vi "Go Back.vi"(0 "Display State In":T1={"WebView2 Ref"=refnum, "event callback refnum"=refnum, "Events"={"Navigation Complete Event"=refnum, "Source Changed Event"=refnum, "Document Title Changed Event"=refnum, "Status Bar Text Changed"=refnum, "Web Message Received"=refnum, "Window Close Requested"=refnum}, "Paths"={"Webview2 Native"=path "C:/Users/kleins/Desktop/webview2/microsoft.web.webview2.1.0.1370.28/build/native", "Edge Application"=path "", "User Data"=path ""}}, 9 "Container State":T3, 11 "error in (no error)":errorcluster) -> (4 "Display State Out":T1={"WebView2 Ref"=refnum, "event callback refnum"=refnum, "Events"={"Navigation Complete Event"=refnum, "Source Changed Event"=refnum, "Document Title Changed Event"=refnum, "Status Bar Text Changed"=refnum, "Web Message Received"=refnum, "Window Close Requested"=refnum}, "Paths"={"Webview2 Native"=path "C:/Users/kleins/Desktop/webview2/microsoft.web.webview2.1.0.1370.28/build/native", "Edge Application"=path "", "User Data"=path ""}}, 15 "error out":errorcluster)   [LabVIEW 2020, in "WebView2 Control.xctl"]
uses:
  WebView2 Control.xctl
  <vilib>/_xctls/Container State.ctl
  State.ctl
  C:/Users/kleins/Desktop/webview2/microsoft.web.webview2.1.0.1370.28/lib/net45/Microsoft.Web.WebView2.WinForms.dll
  microsoft.web.webview2.1.0.1370.28/lib/net45/Microsoft.Web.WebView2.WinForms.dll
  Paths.ctl
  <vilib>/_xctls/XControlSupport.lvlib
panel:
  # "Add Controls & Indicators that form the parameters of the method here. Hook them to the connector pane. Do not delete the controls & indicators that are already hooked to the connector pane.\n \nTo setup the parameters  for this method, right click on this item in the Project Tree & select \"Configure Method...\"."
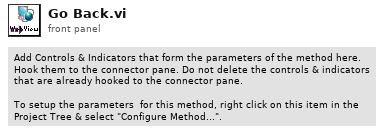
[diagram p1: front panel]
types:
  T1 = typedef "WebView2 Control.xctl/State.ctl" = cluster{"WebView2 Ref":refnum<data-value>, "event callback refnum":refnum<k27>, "Events":cluster{"Navigation Complete Event":refnum<user-event>, "Source Changed Event":refnum<user-event>, "Document Title Changed Event":refnum<user-event>, "Status Bar Text Changed":refnum<user-event>, "Web Message Received":refnum<user-event>, "Window Close Requested":refnum<user-event>}, "Paths":T2}
  T2 = typedef "WebView2 Control.xctl/Paths.ctl" = cluster{"Webview2 Native":path, "Edge Application":path, "User Data":path}
  T3 = typedef "XControlSupport.lvlib/Container State.ctl" = cluster{"Indicator?":bool, "Run Mode?":bool, " Refnum":refnum<vi>}
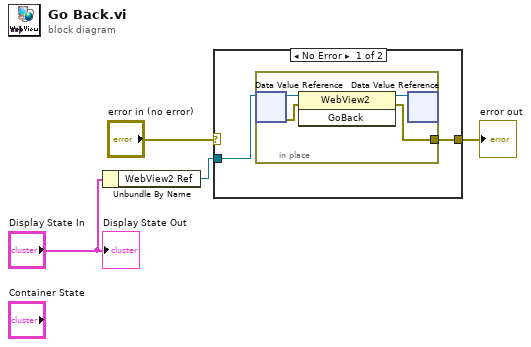
[diagram p0: block diagram]
diagram:
  n1 = Unbundle By Name("Display State In") -> ("WebView2 Ref"=w3:refnum<data-value>)
  n2 = case shown="No Error" "error in (no error)" {
    selector: "error in (no error)" -> [_ w11]
    tunnel: [w6 w11] -> w1
    tunnel: w3 -> [w5 _]
    frame No Error {
      n3 = in-place {
        in-place-border: [w10] -> w6
        n4 = in-place-dvr #1(w5) -> (w9:refnum<k24>, w8:errorcluster)
        n5 = invoke class="WebView2" method="GoBack"(reference=w9, error in=w8) -> (reference out=w7:refnum<k24>, error out=w10:errorcluster)  [unwired: 1 in, 1 out]
        n6 = in-place-dvr #1(w7) -> ()  [unwired: 2 out]
      }
    }
    frame Error {
    }
  }
  "error out" <- w1
  "Display State Out" <- "Display State In"
